vi "search frame pos.vi"(8 "error in (no error)":errorcluster, 10 "Frame Number":u32, 11 "String":string) -> (0 "error out":errorcluster, 1 "Found":bool, 2 "Line Num":i32, 3 "Position":i32)   [LabVIEW 2018, in "Frame Analizer.lvclass"]
uses:
  Frame Analizer.lvclass
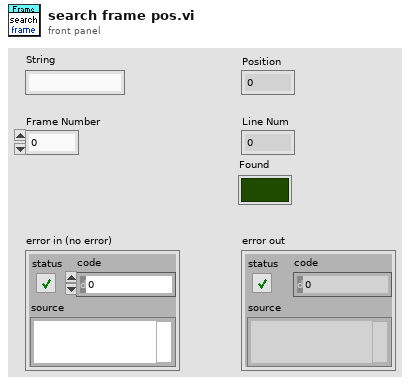
[diagram p1: front panel]
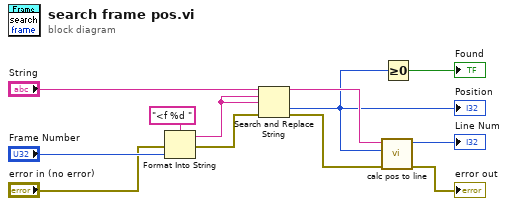
[diagram p0: block diagram]
diagram:
  n1 = Format Into String(format string="<f %d ", error in="error in (no error)", "Frame Number") -> (resulting string=w10:string, error out=w6:errorcluster)  [unwired: 1 in]
  n2 = Search and Replace String(input string="String", search string=w10, replace string=w10, error in=w6) -> (result string=w11:string, offset past replacement=w2:i32, error out=w5:errorcluster)  [unwired: 4 in, 1 out]
  "Position" <- w2
  n3 = call "calc pos to line.vi"("error in (no error)"=w5, "cursor pos"=w2, "String"=w11) -> ("error out"=→"error out":errorcluster, "line num"=→"Line Num":i32)  [unwired: 7 in]
  n4 = Greater Or Equal To 0?(x=w2) -> (x >= 0?=→"Found":bool)
